vi "IsNull.vi"(4 "ProductB":refnum<class "ProductB.lvclass">) -> (1 "isNull":bool)   [LabVIEW 2020, in "FactoryMethod.lvlib" / "FactoryMethodLazyEvaluation.lvlib" / "ProductB.lvclass"]
uses:
  ProductB.lvclass
  ProductB.lvclass/ProductB.ctl
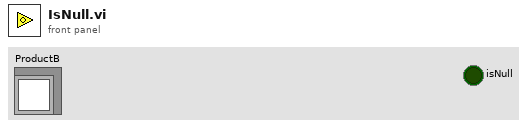
[diagram p1: front panel]
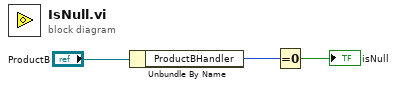
[diagram p0: block diagram]
diagram:
  n1 = Unbundle By Name("ProductB") -> ("ProductBHandler"=w3:u32)
  n2 = Equal To 0?(x=w3) -> (x = 0?=→"isNull":bool)
